vi "test fpga 796xR.vi"() -> ()   [LabVIEW 2015]
uses:
  <vilib>/Platform/TimedLoop/XDataNode/timing_clust.ctl
  <vilib>/Platform/TimedLoop/XDataNode/nitl_modes.ctl
  <vilib>/Platform/TimedLoop/XDataNode/wakeup.ctl
  <vilib>/rvi/Emulation/niFpgaSctlEmulationGetInTimedLoop.vi
  <vilib>/rvi/Emulation/niFpgaEmulationReportErrorSimple.vi
  <vilib>/rvi/Emulation/niFpgaGetClockAttributes.vi
  <vilib>/rvi/Emulation/niFpgaCriticalErrorInLSC.vi
  <vilib>/rvi/eio/common/nirviEmuTemplateMethod_errors.vi
  <vilib>/rvi/interface/RandomDataEmulation/niFpgaRandomDataHandleErrors.vi
  <vilib>/Platform/TimedLoop/XDataNode/XDataNode.xnode
  <vilib>/eio/EIONode/EIONode.xnode
  <vilib>/rvi/DataTransferAndStorage/Container/XNode/niFpgaContainer.xnode
  <vilib>/rvi/interface/RandomDataEmulation/nirviRandomDataFpgaReadWriteTemplate.vi
  <vilib>/Platform/TimedLoop/XDataNode/XDNodeRunTimeDep.lvlib
panel:
  out "数值输入控件":i32
  in  "数组":i16[](array[numeric])
  in  "Microscope":enum16{"Miniature", "Benchtop"}(ring)
  in  "Switch":bool
  out "Acq.Point":i32
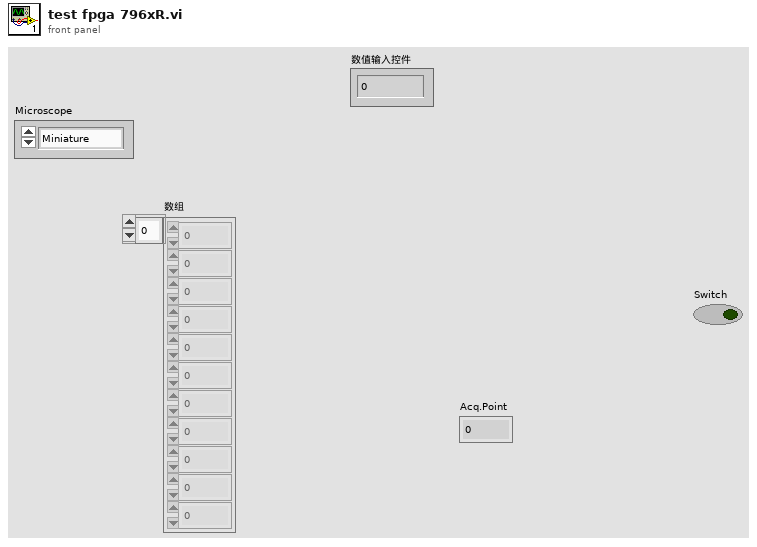
[diagram p1: front panel]
types:
  T1 = typedef "XDNodeRunTimeDep.lvlib/timing_clust.ctl" = cluster{"Expected End [f-1]":u64, "Actual End [f-1]":u64, "Finished Late? [f-1]":bool, "Expected End [i-1]":u64, "Actual End [i-1]":u64, "Finished Late? [i-1]":bool, "Expected Start [i]":u64, "Actual Start [i]":u64, "Expected Start [f]":u64, "Actual Start [f]":u64, "Source Name":string, "Structure Name":string, "Period":i64, "Deadline":i64, "Offset":i64, "Start":i64, "Priority":i32, "Timeout":i32, "Mode":T2, "Wakeup Reason":T3, "Error":errorcluster, "Source Type":string, "Secondary Source Type":string, "Global End Time":u64, "Global Start Time":u64, "Frame Duration":u64, "Iteration Duration":u64, "Assigned CPU":i32, "I/O Scan Engine Mode":u32}
  T2 = typedef "XDNodeRunTimeDep.lvlib/nitl_modes.ctl" = enum32{"No Change", "Process missed periods, maintain original phase", "Discard missed periods, maintain original phase", "Process missed periods, ignore original phase", "Discard missed periods, ignore original phase"}
  T3 = typedef "XDNodeRunTimeDep.lvlib/wakeup.ctl" = enum32{"Normal", "Aborted", "Asynchronous wakeup", "Timing source error", "Timed loop error", "Timeout"}
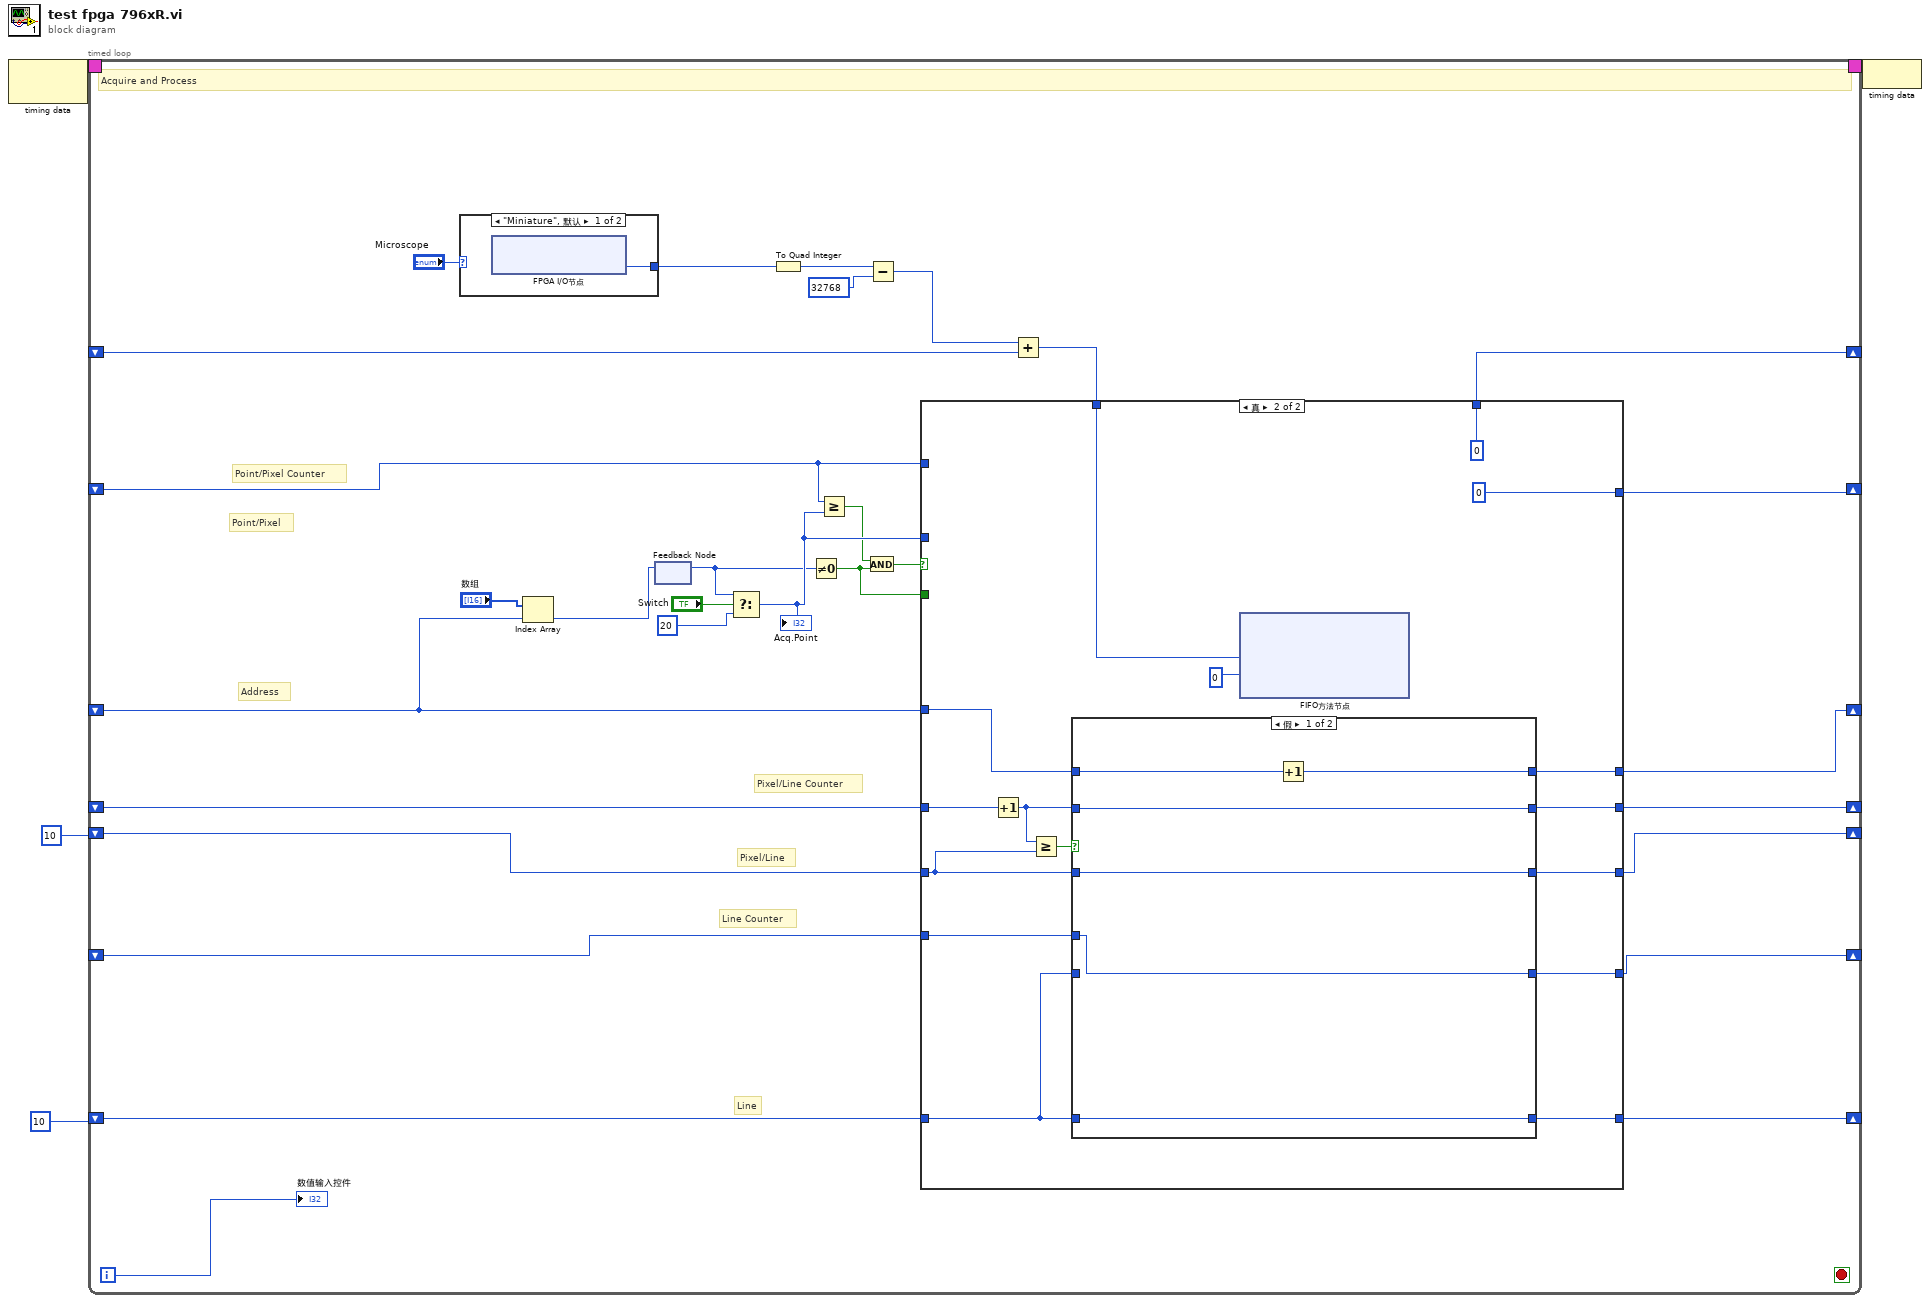
[diagram p0: block diagram]
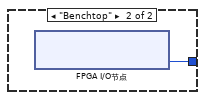
[diagram p2: hidden frame]
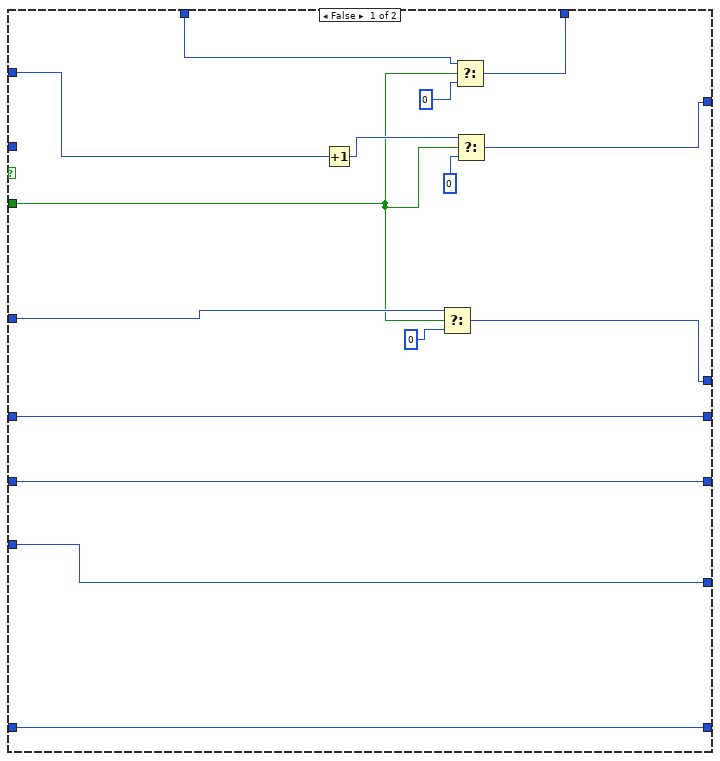
[diagram p3: hidden frame]
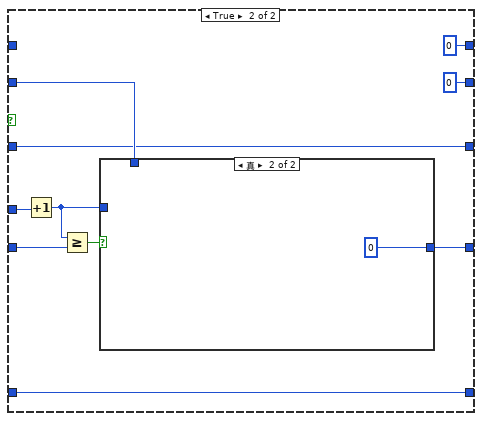
[diagram p4: hidden frame]
diagram:
  n1 = node-c288() -> (w4:T1)  [unwired: 1 in]
  n2 = timed-loop {
    timing: w4 -> [_]
    timing-out: [_] -> w3
    shift-right: [w34] -> _
    shift-left: _ -> [w6]
    shift-right: [w32] -> _
    shift-left: _ -> [w33]
    shift-right: [w30] -> _
    shift-left: _ -> [w31]
    shift-right: [w28] -> _
    shift-left: _ -> [w29]
    shift-right: [w26] -> _
    shift-left: u32 10 ("t") -> [w27]
    shift-right: [w24] -> _
    shift-left: u32 10 ("t") -> [w25]
    shift-right: [w23] -> _
    shift-left: _ -> [w8]
    i -> [w5]
    stop <- _ stop-if-true
    # "Line Counter"
    # "Line"
    # "Pixel/Line Counter"
    # "Pixel/Line"
    # "Address"
    # "Point/Pixel"
    # "Point/Pixel Counter"
    # "Acquire and Process"
    n3 = case shown="\"Miniature\", 默认" "Microscope" {
      tunnel: [w35 w36] -> w15
      frame "Miniature", Default {
        n4 = xnode "FPGA I/O节点"() -> ("IO Module\\AI 0"=w35:u16)  [unwired: 1 in, 1 out]
      }
      frame "Benchtop" {
        n5 = xnode "FPGA I/O节点"() -> ("IO Module\\AI 1"=w36:u16)  [unwired: 1 in, 1 out]
      }
    }
    n6 = Index Array(array="数组", index=w8) -> (element=w7:i16)
    n7 = feedback #1 ("反馈节点")() -> (w14:i16)  [unwired: 1 in]
    n8 = feedback-in #1(w7) -> ()
    n9 = Select(t=w14, s="Switch", f=u32 20 ("t")) -> (s? t:f=w16:u32)
    "Acq.Point" <- w16
    n10 = To Quad Integer(1:w15) -> (0:w19:i64)
    n11 = Not Equal To 0?(x=w14) -> (x != 0?=w11:bool)
    n12 = Greater Or Equal?(x=w6, y=w16) -> (x >= y?=w13:bool)
    n13 = And(x=w13, y=w11) -> (x .and. y?=w12:bool)
    n14 = Subtract(x=w19, y=i64 32768) -> (x-y=w20:i64)
    n15 = Add(x=w20, y=w31) -> (x+y=w22:i64)
    n16 = case shown="真" w12 {
      tunnel: w22 -> [w37 w54]
      tunnel: [w45 i64 0 ("x")] -> w30
      tunnel: [w46 0 ("t")] -> w34
      tunnel: w33 -> [w49 w61]
      tunnel: w29 -> [w48 w65]
      tunnel: [w48 w64] -> w28
      tunnel: [w49 w60] -> w32
      tunnel: w25 -> [w51 w62]
      tunnel: [w50 w53] -> w26
      tunnel: w27 -> [w50 w52]
      tunnel: [w51 w63] -> w24
      tunnel: w8 -> [w40 w59]
      tunnel: [w44 w58] -> w23
      tunnel: w16 -> [_ _]
      tunnel: w6 -> [w47 _]
      tunnel: w11 -> [w39 _]
      frame False {
        n17 = Increment(x=w47) -> (x+1=w42:u32)
        n18 = Select(t=w40, s=w39, f=u32 0 ("t")) -> (s? t:f=w44:u32)
        n19 = Select(t=w37, s=w39, f=u32 0 ("t")) -> (s? t:f=w45:i64)
        n20 = Select(t=w42, s=w39, f=u32 0 ("t")) -> (s? t:f=w46:u32)
      }
      frame True {
        n21 = Increment(x=w61) -> (x+1=w57:u16)
        n22 = Greater Or Equal?(x=w57, y=w52) -> (x >= y?=w56:bool)
        n23 = case shown="假" w56 {
          tunnel: w65 -> [w71 w83]
          tunnel: [w71 w82] -> w64
          tunnel: w62 -> [_ w74]
          tunnel: [w73 w79] -> w63
          tunnel: w62 -> [w73 w79]
          tunnel: [w72 u16 0] -> w60
          tunnel: w57 -> [w72 w77]
          tunnel: w59 -> [w70 _]
          tunnel: [w69 u32 0] -> w58
          tunnel: [w68 w75] -> w53
          tunnel: w52 -> [w68 w75]
          frame False {
            n24 = Increment(x=w70) -> (x+1=w69:u32)
          }
          frame True {
            n25 = Increment(x=w83) -> (x+1=w80:u16)
            n26 = Greater Or Equal?(x=w80, y=w74) -> (x >= y?=w81:bool)
            n27 = case shown="真" w81 {
              tunnel: w80 -> [w84 _]
              tunnel: [w84 u16 0] -> w82
              tunnel: w77 -> [_ _]
              frame False {
              }
              frame True {
              }
            }
          }
        }
        n28 = xnode ("FIFO方法节点")("元素"=w54, "超时"=0) -> ()  [unwired: 1 in, 2 out]
      }
    }
    "数值输入控件" <- w5
  }
  n29 = node-c288(w3) -> ()
